vi "openPictureFile.vi"(8 "error in (no error)":errorcluster, 11 "xwpfRun.Figure in":refnum<class "xwpfRun.Figure.lvclass">) -> (0 "error out":errorcluster, 3 "xwpfRun.Figure out":refnum<class "xwpfRun.Figure.lvclass">)   [LabVIEW 2017, in "Word_Specific.lvlib" / "xwpfRun.Figure.lvclass"]
uses:
  xwpfRun.Figure.lvclass
  xwpfRun.Figure.lvclass/xwpfRun.Figure.ctl
  Support/File Stream/File Stream.lvlib
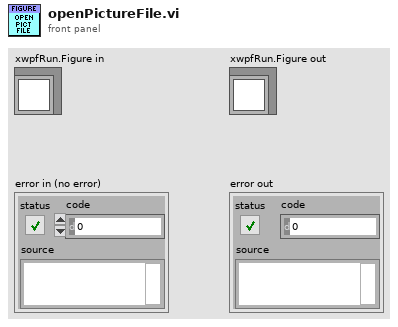
[diagram p1: front panel]
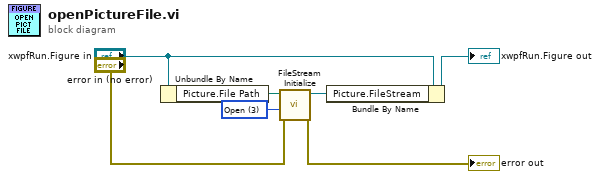
[diagram p0: block diagram]
diagram:
  w1 = 3 items=["CreateNew"=1, "Create"=2, "Open"=3, "OpenOrCreate"=4, "Truncate"=5, "Append"=6] ("mode")
  n1 = Unbundle By Name("xwpfRun.Figure in") -> ("Picture.File Path"=w2:path)
  n2 = call "FileStream Initialize.vi"("error in (no error)"="error in (no error)", "mode"=w1, "path"=w2) -> ("error out"=→"error out":errorcluster, "new reference"=w7:refnum<k24>)  [unwired: 7 in]
  n3 = Bundle By Name(cluster="xwpfRun.Figure in", "Picture.FileStream"=w7) -> (→"xwpfRun.Figure out":refnum<class "xwpfRun.Figure.lvclass">)
